vi "Read tipo_generador.vi"(8 "error in (no error)":errorcluster, 11 "AjustesPrevios in":refnum<class "AjustesPrevios.lvclass">) -> (0 "error out":errorcluster, 2 "tipo_generador":string, 3 "AjustesPrevios out":refnum<class "AjustesPrevios.lvclass">)   [LabVIEW 2019, in "AjustesPrevios.lvclass"]
uses:
  AjustesPrevios.lvclass
  AjustesPrevios.lvclass/AjustesPrevios.ctl
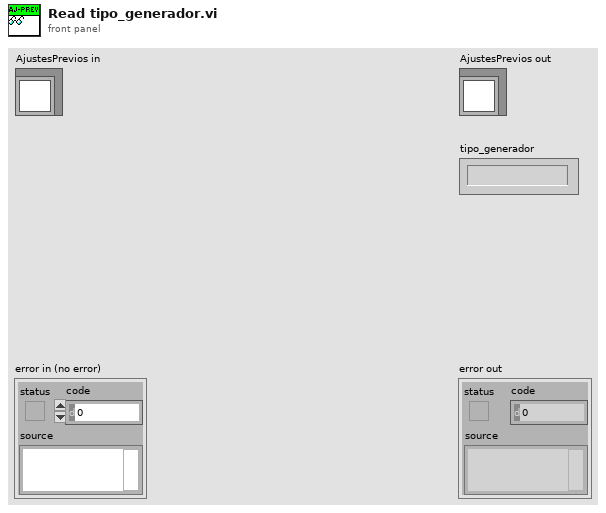
[diagram p1: front panel]
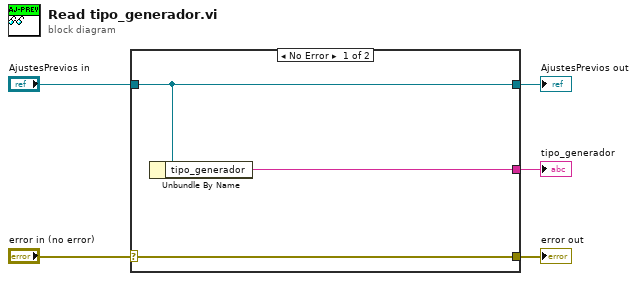
[diagram p0: block diagram]
diagram:
  n1 = case shown="No Error" "error in (no error)" {
    selector: "error in (no error)" -> [w8 w9]
    tunnel: [w8 w9] -> w4
    tunnel: [w7 w10] -> w2
    tunnel: "AjustesPrevios in" -> [w7 w10]
    tunnel: [w6 _] -> w1
    frame No Error {
      n2 = Unbundle By Name(w7) -> ("tipo_generador"=w6:string)
    }
    frame Error {
    }
  }
  "error out" <- w4
  "AjustesPrevios out" <- w2
  "tipo_generador" <- w1
